vi "Autonomous.vi"   [LabVIEW 2017]
doc: "This VI starts when autonomous period begins, and will automatically be terminated when it ends. You can carry out timed or sensor driven operations directly to I/O or to subsystems without needing to return to the caller."
uses:
  <vilib>/Rock Robotics/WPI/Utilities/WPI_GetSetVariantRefNum.vi
  <vilib>/Rock Robotics/Network Tables/NT Read String.vi
  <vilib>/Rock Robotics/Network Tables/NT Write Boolean.vi
  Framework/Robot Global Data.vi
types:
  T1 = typedef "WPI_DriverStationAllianceInfo.ctl" = enum16{"Red", "Blue", "Invalid"}
  T2 = typedef "WPI_JoystickDevRef.ctl" = cluster{"Device":T3}
  T3 = typedef "WPI_JoystickDeviceEnum.ctl" = enum16{"USB 0", "USB 1", "USB 2", "USB 3", "USB 4", "USB 5"}
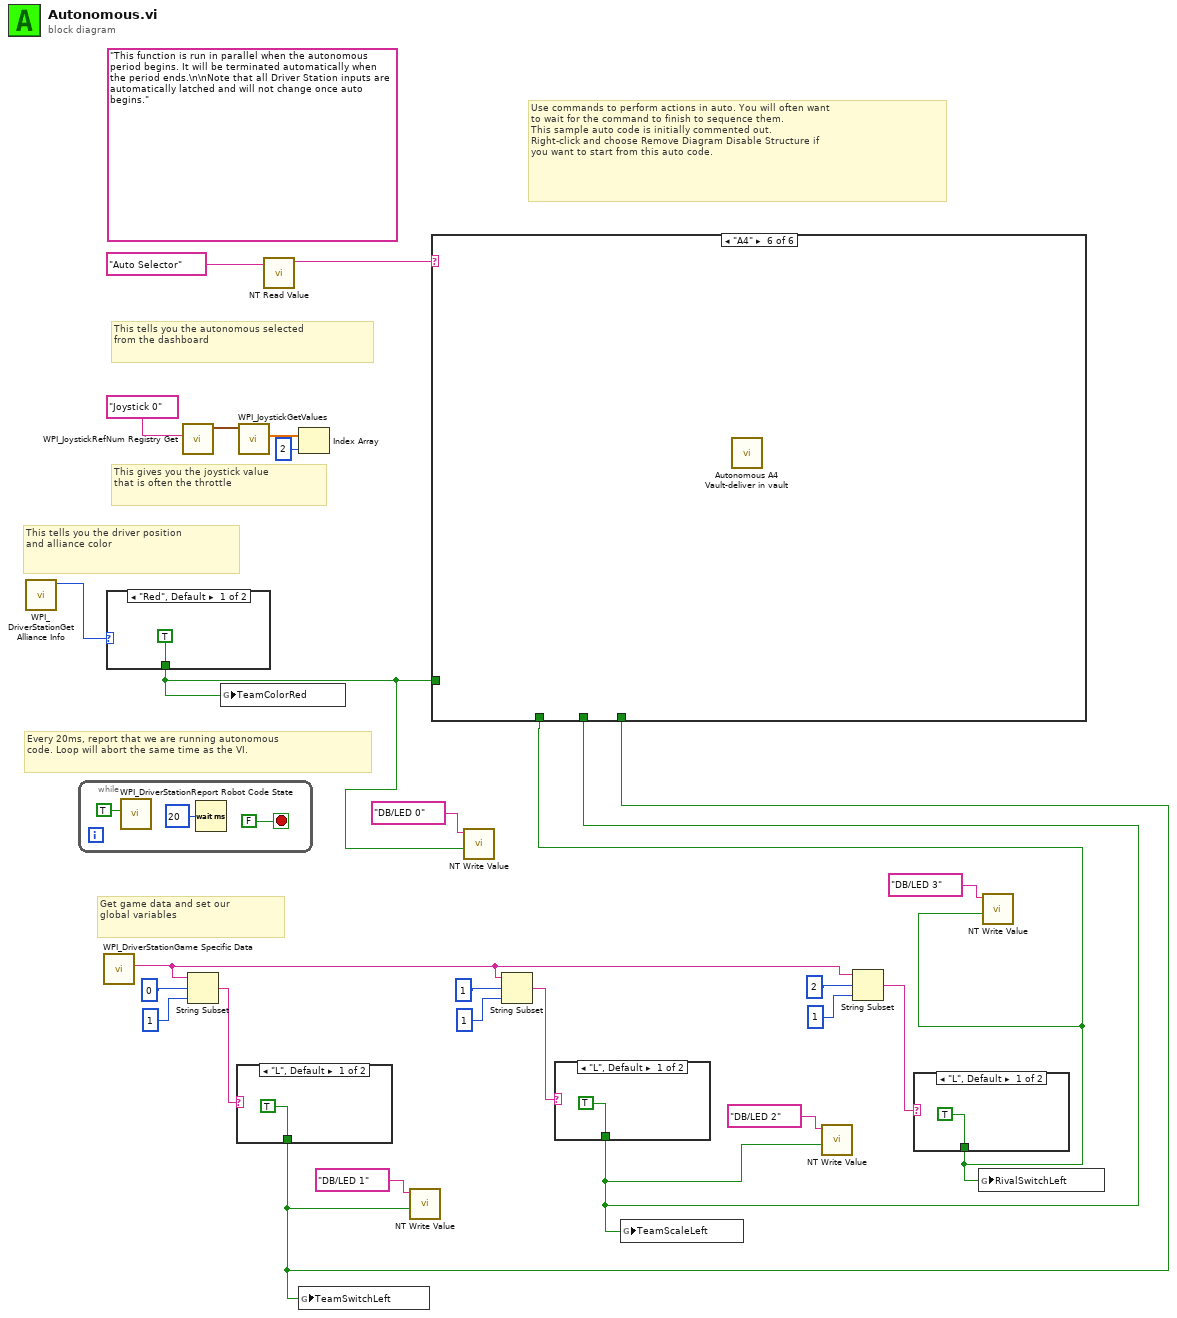
[diagram p0: block diagram]
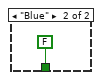
[diagram p2: hidden frame]
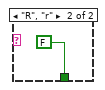
[diagram p3: hidden frame]
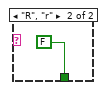
[diagram p4: hidden frame]
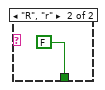
[diagram p5: hidden frame]
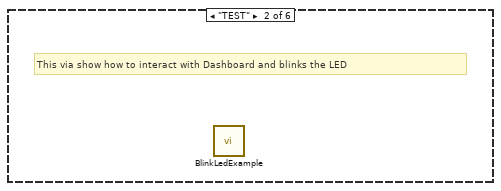
[diagram p7: hidden frame]
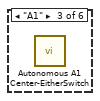
[diagram p8: hidden frame]
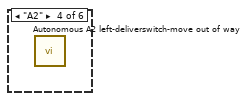
[diagram p9: hidden frame]
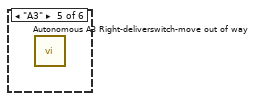
[diagram p10: hidden frame]
diagram:
  (unwired) "This function is run in parallel when the autonomous period begins. It will be terminated automatically when the period ends.\n\nNote that all Driver Station inputs are automatically latched and will not change once auto begins."
  # "Get game data and set our \nglobal variables"
  # "This tells you the autonomous selected\nfrom the dashboard"
  # "Every 20ms, report that we are running autonomous\ncode. Loop will abort the same time as the VI."
  # "This gives you the joystick value\nthat is often the throttle"
  # "Use commands to perform actions in auto. You will often want\nto wait for the command to finish to sequence them.\nThis sample auto code is initially commented out. \nRight-click and choose Remove Diagram Disable Structure if\nyou want to start from this auto code."
  # "This tells you the driver position\nand alliance color"
  n1 = call <vilib>:"WPI_DriverStationGet Alliance Info.vi"() -> ("Alliance"=w9:T1)  [unwired: 11 out]
  n2 = while {
    stop <- FALSE stop-if-true
    n3 = call <vilib>:"WPI_DriverStationReport Robot Code State.vi"("Autonomous"=TRUE) -> ()  [unwired: 10 in, 1 out]
    n4 = Wait (ms)(milliseconds to wait=u32 20) -> ()  [unwired: 1 out]
  }
  n5 = call <vilib>:"WPI_DriverStationGame Specific Data.vi"() -> ("Game Specific Data"=w13:string)  [unwired: 11 in]
  n6 = case shown="\"Red\", Default" w9 {
    tunnel: [TRUE FALSE] -> w1
    frame "Red", Default {
    }
    frame "Blue" {
    }
  }
  n7 = call <vilib>:"WPI_JoystickRefNum Registry Get.vi"("refnum name"="Joystick 0") -> ("JoystickDevRef"=w24:T2)  [unwired: 1 in, 9 out]
  n8 = String Subset(string=w13, offset (0)=0, length (rest)=1 ("length (rest)")) -> (substring=w12:string)
  n9 = global write "Robot Global Data.vi" "TeamColorRed"(w1) -> ()
  n10 = case shown="\"L\", Default" w12 {
    tunnel: [TRUE FALSE] -> w2
    frame "L", Default {
    }
    frame "R", "r" {
    }
  }
  n11 = call <vilib>:"WPI_JoystickGetValues.vi"("JoystickDevRef"=w24) -> ("Axes"=w23:dbl[])  [unwired: 6 in, 4 out]
  n12 = call-poly <vilib>:"NT Read Value.vi"("Name"="Auto Selector") -> ("String"=w20:string)  [unwired: 9 in, 1 out]
  n13 = Index Array(array=w23, index=2) -> ()  [unwired: 1 out]
  n14 = global write "Robot Global Data.vi" "TeamSwitchLeft"(w2) -> ()
  n15 = call-poly <vilib>:"NT Write Value.vi"("Boolean"=w2, "Name"="DB/LED 1") -> ()  [unwired: 9 in, 1 out]
  n16 = call-poly <vilib>:"NT Write Value.vi"("Boolean"=w1, "Name"="DB/LED 0") -> ()  [unwired: 9 in, 1 out]
  n17 = String Subset(string=w13, offset (0)=1, length (rest)=1 ("length (rest)")) -> (substring=w11:string)
  n18 = case shown="\"L\", Default" w11 {
    tunnel: [TRUE FALSE] -> w3
    frame "L", Default {
    }
    frame "R", "r" {
    }
  }
  n19 = global write "Robot Global Data.vi" "TeamScaleLeft"(w3) -> ()
  n20 = call-poly <vilib>:"NT Write Value.vi"("Boolean"=w3, "Name"="DB/LED 2") -> ()  [unwired: 9 in, 1 out]
  n21 = String Subset(string=w13, offset (0)=2, length (rest)=1 ("length (rest)")) -> (substring=w10:string)
  n22 = case shown="\"L\", Default" w10 {
    tunnel: [TRUE FALSE] -> w4
    frame "L", Default {
    }
    frame "R", "r" {
    }
  }
  n23 = case shown="\"A4\"" w20 {
    tunnel: w1 -> [_ _ _ _ _ _]
    tunnel: w4 -> [_ _ _ _ _ _]
    tunnel: w3 -> [_ _ _ _ _ _]
    tunnel: w2 -> [_ _ _ _ _ _]
    frame Default {
      # "You can put your main auto here, or you can right-click on the case and make any\nother frame be the default case."
      # "This is the frame that will execute if no selection is made, or if it is not recognized"
    }
    frame "TEST" {
      # "This via show how to interact with Dashboard and blinks the LED"
      n24 = call "BlinkLedExample.vi"() -> ()  [unwired: 12 in]
    }
    frame "A1" {
      n25 = call "Autonomous A1 Center-EitherSwitch.vi"() -> ()  [unwired: 12 in]
    }
    frame "A2" {
      n26 = call "Autonomous A2 left-deliverswitch-move out of way.vi"() -> ()  [unwired: 16 in]
    }
    frame "A3" {
      n27 = call "Autonomous A3 Right-deliverswitch-move out of way.vi"() -> ()  [unwired: 12 in]
    }
    frame "A4" {
      n28 = call "Autonomous A4 Vault-deliver in vault.vi"() -> ()  [unwired: 12 in]
    }
  }
  n29 = global write "Robot Global Data.vi" "RivalSwitchLeft"(w4) -> ()
  n30 = call-poly <vilib>:"NT Write Value.vi"("Boolean"=w4, "Name"="DB/LED 3") -> ()  [unwired: 9 in, 1 out]
